vi "Log Framework Event.vi"(7 "Event Level (Debug)":T1, 8 "error in (no error)":errorcluster, 9 "Data To Log":string, 11 "IObserver in":refnum<class "IObserver.lvclass">) -> (0 "error out":errorcluster)   [LabVIEW 2020, in "IObserver.lvlib" / "IObserver.lvclass"]
doc: "日志框架事件"
uses:
  IObserver.lvclass
  composed-event-logger/Source/Composed Log/Types/Log Level.ctl
  IObserver.lvclass/IObserver.ctl
  composed-event-logger/Source/Composed Log/LoggerReference/LoggerReference.lvclass/LoggerReference.ctl
  composed-event-logger/Source/Composed Log/LoggerReference/Log.vi
  composed-event-logger/Source/Composed Log/LoggerReference/Get Valid Event Time.vi
  composed-event-logger/Source/Composed Log/LoggerReference/Remove Stale Logs.vi
  composed-event-logger/Source/Composed Log/LoggerReference/LoggerReference.lvclass
  composed-event-logger/Source/Composed Log/Composed Log.lvlib
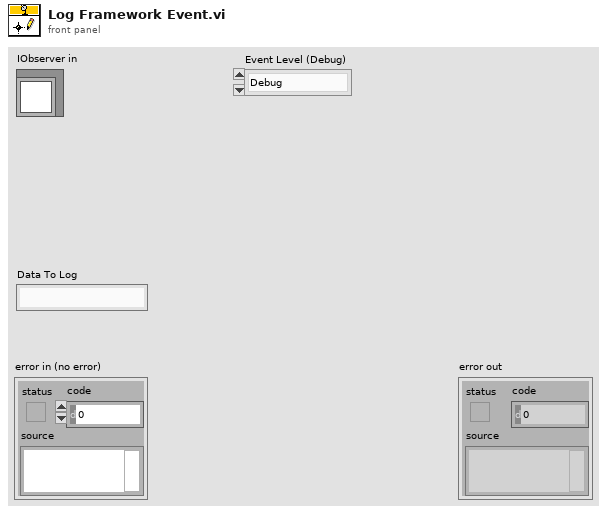
[diagram p1: front panel]
types:
  T1 = typedef "Composed Log.lvlib/Log Level.ctl" = enum16{"Debug", "Info", "Warning", "Error", "Critical"}
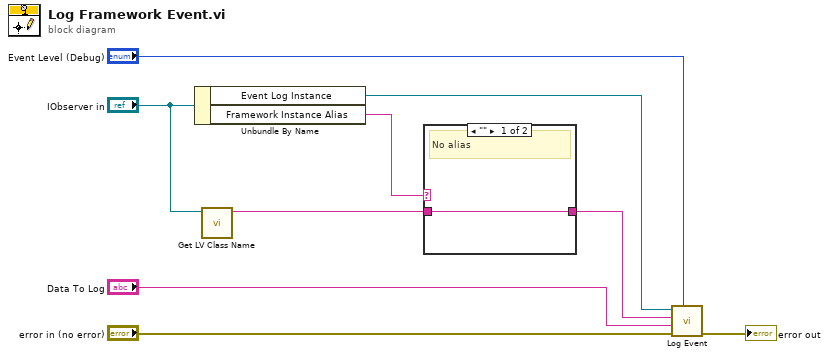
[diagram p0: block diagram]
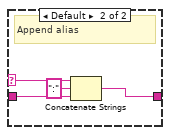
[diagram p2: hidden frame]
diagram:
  n1 = Unbundle By Name("IObserver in") -> ("Event Log Instance"=w7:refnum<class "LoggerReference.lvclass">, "Framework Instance Alias"=w5:string)
  n2 = call <vilib>:"Get LV Class Name.vi"("object"="IObserver in") -> ("class name"=w2:string)  [unwired: 9 in, 1 out]
  n3 = case shown="\"\"" w5 {
    selector: w5 -> [_ w14]
    tunnel: [w10 w13] -> w4
    tunnel: w2 -> [w10 w12]
    frame "" {
      # "No alias"
    }
    frame Default {
      # "Append alias"
      n4 = Concatenate Strings(w14, ":" ("string"), w12) -> (w13:string)
    }
  }
  n5 = call "Log Event.vi"("Event Level"="Event Level (Debug)", "error in (no error)"="error in (no error)", "Data To Log"="Data To Log", "SourceID"=w4, "Log Instance"=w7) -> ("error out"=→"error out":errorcluster)  [unwired: 5 in, 1 out]
